vi "write binary.vi"(10 "binary":string, 11 "websocket client in":refnum<class "websocket client.lvclass">) -> (0 "error out":errorcluster, 3 "websocket client out":refnum<class "websocket client.lvclass">)   [LabVIEW 2016, in "websocket client.lvclass"]
uses:
  websocket client.lvclass
  opcode.ctl
  websocket client.lvclass/websocket client.ctl
  websocket core.lvlib
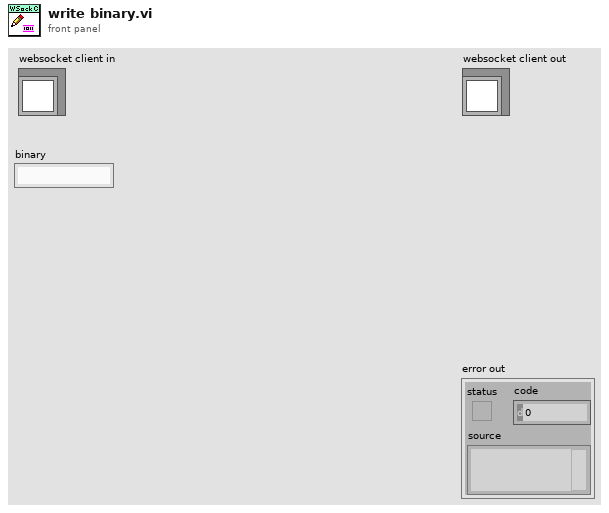
[diagram p1: front panel]
types:
  T1 = typedef "websocket core.lvlib/opcode.ctl" = u8
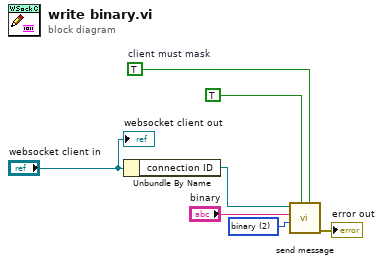
[diagram p0: block diagram]
diagram:
  w1 = TRUE  # client must mask
  w4 = T1 2 items=["text"=1, "binary"=2, "x3"=3, "x4"=4, "x5"=5, "x6"=6, "x7"=7] ("opcode")
  n1 = Unbundle By Name("websocket client in") -> ("connection ID"=w6:refnum<k5>)
  n2 = call "send message.vi"("mask? (F)"=w1, "final fragment (T)"=TRUE, "opcode"=w4, "data"="binary", "TCP Network Connection in"=w6) -> ("error out"=→"error out":errorcluster)  [unwired: 6 in]
  "websocket client out" <- "websocket client in"
